vi "retrieveConfiguration.vi"(8 "error in (no error)":errorcluster, 10 "dataName":string, 11 "Target in":refnum<class "Target.lvclass">) -> (0 "error out":errorcluster, 2 "dataValueFromFile":string, 3 "Target out":refnum<class "Target.lvclass">)   [LabVIEW 2012, in "Target.lvclass"]
doc: "Retrieves the configuration data from the file associated with dataName."
uses:
  Target.lvclass
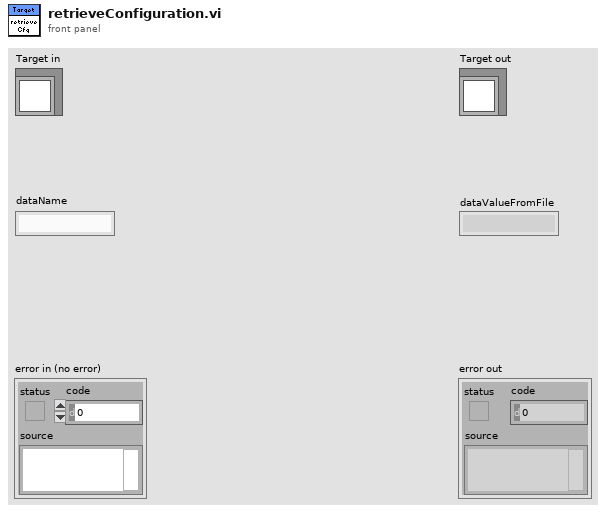
[diagram p1: front panel]
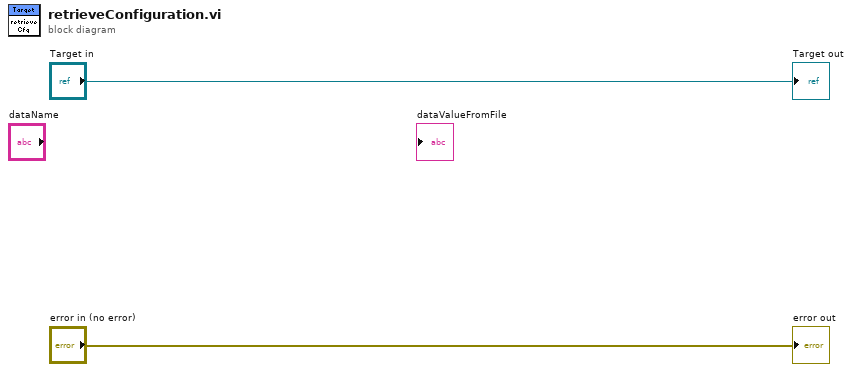
[diagram p0: block diagram]
diagram:
  "error out" <- "error in (no error)"
  "Target out" <- "Target in"
